vi "Change to Position Control.vi"(0 "Jag ID":i8, 1 "P":dbl, 2 "I":dbl, 3 "D":dbl, 4 "Jag Refnum Name":string) -> (5 "MotorControlDevRef":T1={"DeviceStatus"={"status"=FALSE, "code"=0, "source"=""}, "Type"=enum."PWM", "PWM"={"Digital Module"=enum."Digital Module 1", "PWM Channel"=enum."Invalid", "DeadBand"={"Name"="", "maxPositivePwm"=0, "minPositivePwm"=0, "centerPwm"=0, "maxNegativePwm"=0, "minNegativePwm"=0, "angularRange"=0}}, "CAN"={"Device Number"=0, "Control Mode"=enum."Percent VBus", "Semaphore"=refnum, "Max Vout"=12.0}, "Invert"=FALSE, "TransformRef"=refnum, "InvTransformRef"=refnum})   [LabVIEW 2011]
uses:
  <vilib>/Rock Robotics/WPI/MotorControl/WPI_MotorControlDeviceRef.ctl
  <vilib>/Rock Robotics/SystemInterfaces/Typedef/FPGA_TypedefDigitalModule.ctl
  <vilib>/Rock Robotics/SystemInterfaces/DIO/FPGA_DIOPWMChannel.ctl
  <vilib>/Rock Robotics/WPI/PWM/WPI_PWMDeadband.ctl
  <vilib>/Rock Robotics/WPI/CAN/Jaguar/SubVIs/WPI_CANJaguar_ControlMode.ctl
  <vilib>/Rock Robotics/WPI/PWM/WPI_PWMTransform_ConPane.ctl
  <vilib>/Rock Robotics/WPI/CAN/Jaguar/SubVIs/WPI_CANJaguar_PositionReference.ctl
  <vilib>/Rock Robotics/WPI/CAN/Jaguar/SubVIs/WPI_CANJaguar_BrakeCoastMode.ctl
  <vilib>/Rock Robotics/WPI/CAN/Jaguar/SubVIs/WPI_CANJaguar_LimitMode.ctl
  <vilib>/Rock Robotics/WPI/MotorControl/WPI_MotorControlOpenCANJaguar.vi
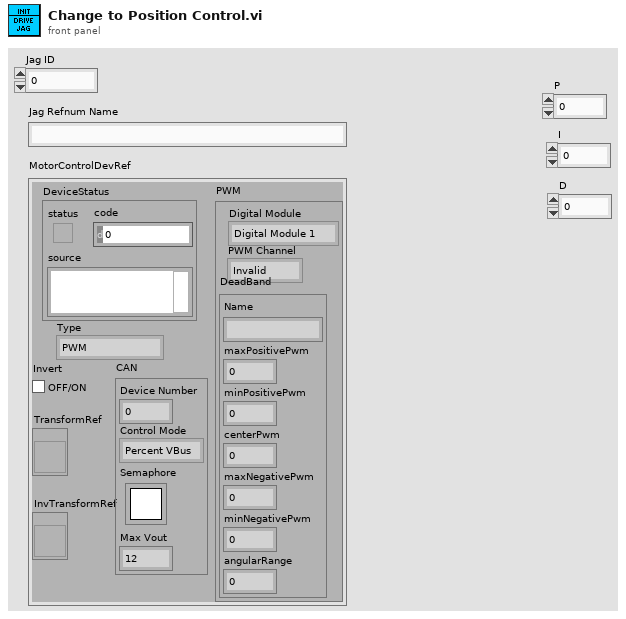
[diagram p1: front panel]
types:
  T1 = typedef "WPI_MotorControlDeviceRef.ctl" = cluster{"DeviceStatus":errorcluster, "Type":enum16{"PWM", "CAN"}, "PWM":cluster{"Digital Module":T2, "PWM Channel":T3, "DeadBand":T4}, "CAN":cluster{"Device Number":u8, "Control Mode":T5, "Semaphore":T6, "Max Vout":dbl}, "Invert":bool, "TransformRef":T7, "InvTransformRef":T7}
  T2 = typedef "FPGA_TypedefDigitalModule.ctl" = enum16{"Digital Module 1", "Digital Module 2"}
  T3 = typedef "FPGA_DIOPWMChannel.ctl" = enum8{"PWM 1", "PWM 2", "PWM 3", "PWM 4", "PWM 5", "PWM 6", "PWM 7", "PWM 8", "PWM 9", "PWM 10", "Invalid"}
  T4 = typedef "WPI_PWMDeadband.ctl" = cluster{"Name":string, "maxPositivePwm":i32, "minPositivePwm":i32, "centerPwm":i32, "maxNegativePwm":i32, "minNegativePwm":i32, "angularRange":u16}
  T5 = typedef "WPI_CANJaguar_ControlMode.ctl" = enum8{"Percent VBus", "Current", "Speed", "Position", "Voltage"}
  T6 = typedef "Semaphore RefNum" = refnum<k1>
  T7 = typedef "WPI_PWMTransform_ConPane.ctl" = refnum<vi>
  T8 = typedef "WPI_CANJaguar_LimitMode.ctl" = enum16{"Switch Inputs Only", "Soft Position Limits"}
  T9 = typedef "WPI_CANJaguar_BrakeCoastMode.ctl" = enum8{"Jumper", "Brake", "Coast"}
  T10 = typedef "WPI_CANJaguar_PositionReference.ctl" = u8
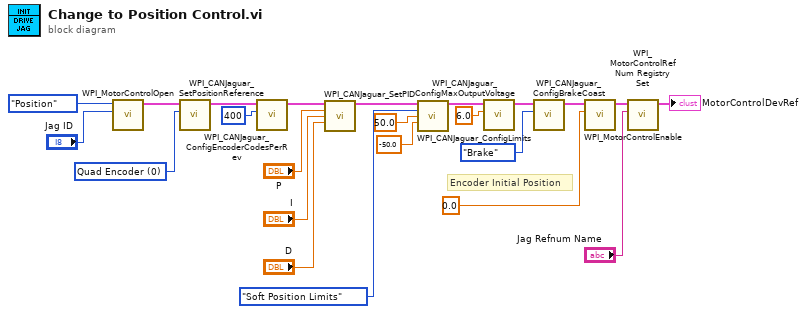
[diagram p0: block diagram]
diagram:
  w10 = T10 0 items=["Quad Encoder"=0, "Potentiometer"=1, "None"=255] ("Position Reference")
  # "Encoder Initial Position"
  n1 = call-poly <vilib>:"WPI_MotorControlOpen.vi"("Device Number"="Jag ID", "Control Mode"=WPI_CANJaguar_ControlMode."Position") -> ("MotorControlDeviceRef"=w17:T1)  [unwired: 8 in, 1 out]
  n2 = call <vilib>:"WPI_CANJaguar_SetPositionReference.vi"("Position Reference"=w10, "CAN Jaguar Ref"=w17) -> ("CAN Jaguar Ref Out"=w16:T1)  [unwired: 8 in, 1 out]
  n3 = call <vilib>:"WPI_CANJaguar_ConfigEncoderCodesPerRev.vi"("Encoder Codes Per Rev"=u16 400, "CAN Jaguar Ref"=w16) -> ("CAN Jaguar Ref Out"=w14:T1)  [unwired: 8 in, 1 out]
  n4 = call <vilib>:"WPI_CANJaguar_SetPID.vi"("CAN Jaguar Ref"=w14, "P"="P", "I"="I", "D"="D") -> ("CAN Jaguar Ref Out"=w9:T1)  [unwired: 10 in, 1 out]
  n5 = call <vilib>:"WPI_CANJaguar_ConfigLimits.vi"("CAN Jaguar Ref"=w9, "Limit Mode"=WPI_CANJaguar_LimitMode."Soft Position Limits", "Forward Limit Position"=50.0, "Reverse Limit Position"=-50.0) -> ("CAN Jaguar Ref Out"=w8:T1)  [unwired: 10 in, 1 out]
  n6 = call <vilib>:"WPI_CANJaguar_ConfigMaxOutputVoltage.vi"("Maximum Output Voltage"=6.0, "CAN Jaguar Ref"=w8) -> ("CAN Jaguar Ref Out"=w7:T1)  [unwired: 8 in, 1 out]
  n7 = call <vilib>:"WPI_CANJaguar_ConfigBrakeCoast.vi"("Brake / Coast Mode"=WPI_CANJaguar_BrakeCoastMode."Brake", "CAN Jaguar Ref"=w7) -> ("CAN Jaguar Ref Out"=w6:T1)  [unwired: 8 in, 1 out]
  n8 = call <vilib>:"WPI_MotorControlEnable.vi"("Encoder Initial Position"=0.0, "CAN Jaguar Ref"=w6) -> ("CAN Jaguar Ref Out"=w22:T1)  [unwired: 8 in, 1 out]
  n9 = call <vilib>:"WPI_MotorControlRefNum Registry Set.vi"("refnum name"="Jag Refnum Name", "MotorControlDevRef"=w22) -> ("MotorControlDevRef"=→"MotorControlDevRef":T1)  [unwired: 8 in, 1 out]
